vi "iBeam Laser Engine.vi"(0 "iBeam Laser Notifier":string, 11 "COM Port":string[](array[string])) -> ()   [LabVIEW 2016]
uses:
  Laser Controls/Laser Notifier Element.ctl
  Laser Controls/Laser Actions.ctl
  Laser Controls/Laser Settings.ctl
  Laser Controls/Laser Parameters.ctl
  Laser Controls/Laser Status.ctl
  <vilib>/Instr/_visa.llb/VISA Configure Serial Port (Instr).vi
panel:
  in  "Get Status":bool
  in  "Get Power":bool
  out "Laser Status":string
  out "Power (uW)":string
  out "Startup Error":errorcluster
  in  "Quit":bool
  in  "Enable Ext":bool
  in  "Laser Power (mW)":dbl
  in  "Laser On/Off":bool
  out "Serial Number":string
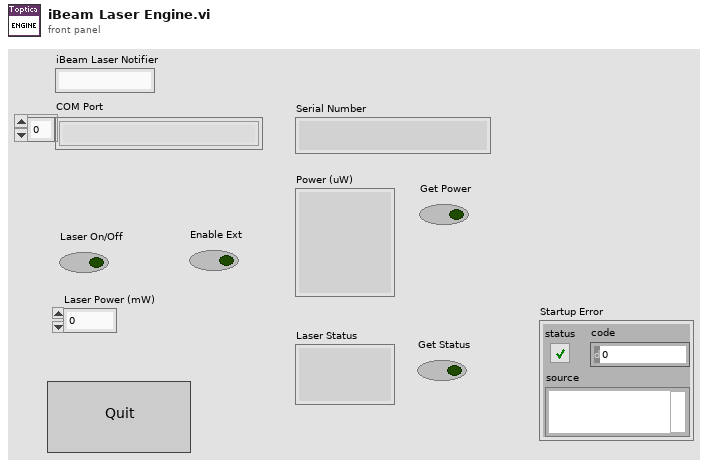
[diagram p1: front panel]
types:
  T1 = typedef "Laser Notifier Element.ctl" = cluster{"Laser Action":T2, "Received?":bool, "Enabled (Interlock)?":bool, "Light Emission?":bool, "Power (mW)":dbl, "Settings":T3, "Status":T5, "Error":errorcluster}
  T2 = typedef "Laser Actions.ctl" = enum16{"Error Check", "Set On/Off", "Set Power", "Set Parameter", "Get Power", "Get Status", "Get Parameter", "Quit"}
  T3 = typedef "Laser Settings.ctl" = cluster{"Laser Parameters":T4, "Value":dbl}
  T4 = typedef "Laser Parameters.ctl" = enum16{"Wavelength (nm)", "Pulsing?", "Rep. Rate", "External Control"}
  T5 = typedef "Laser Status.ctl" = enum16{"Warmup", "Ready", "Emission", "Tuning", "Error"}
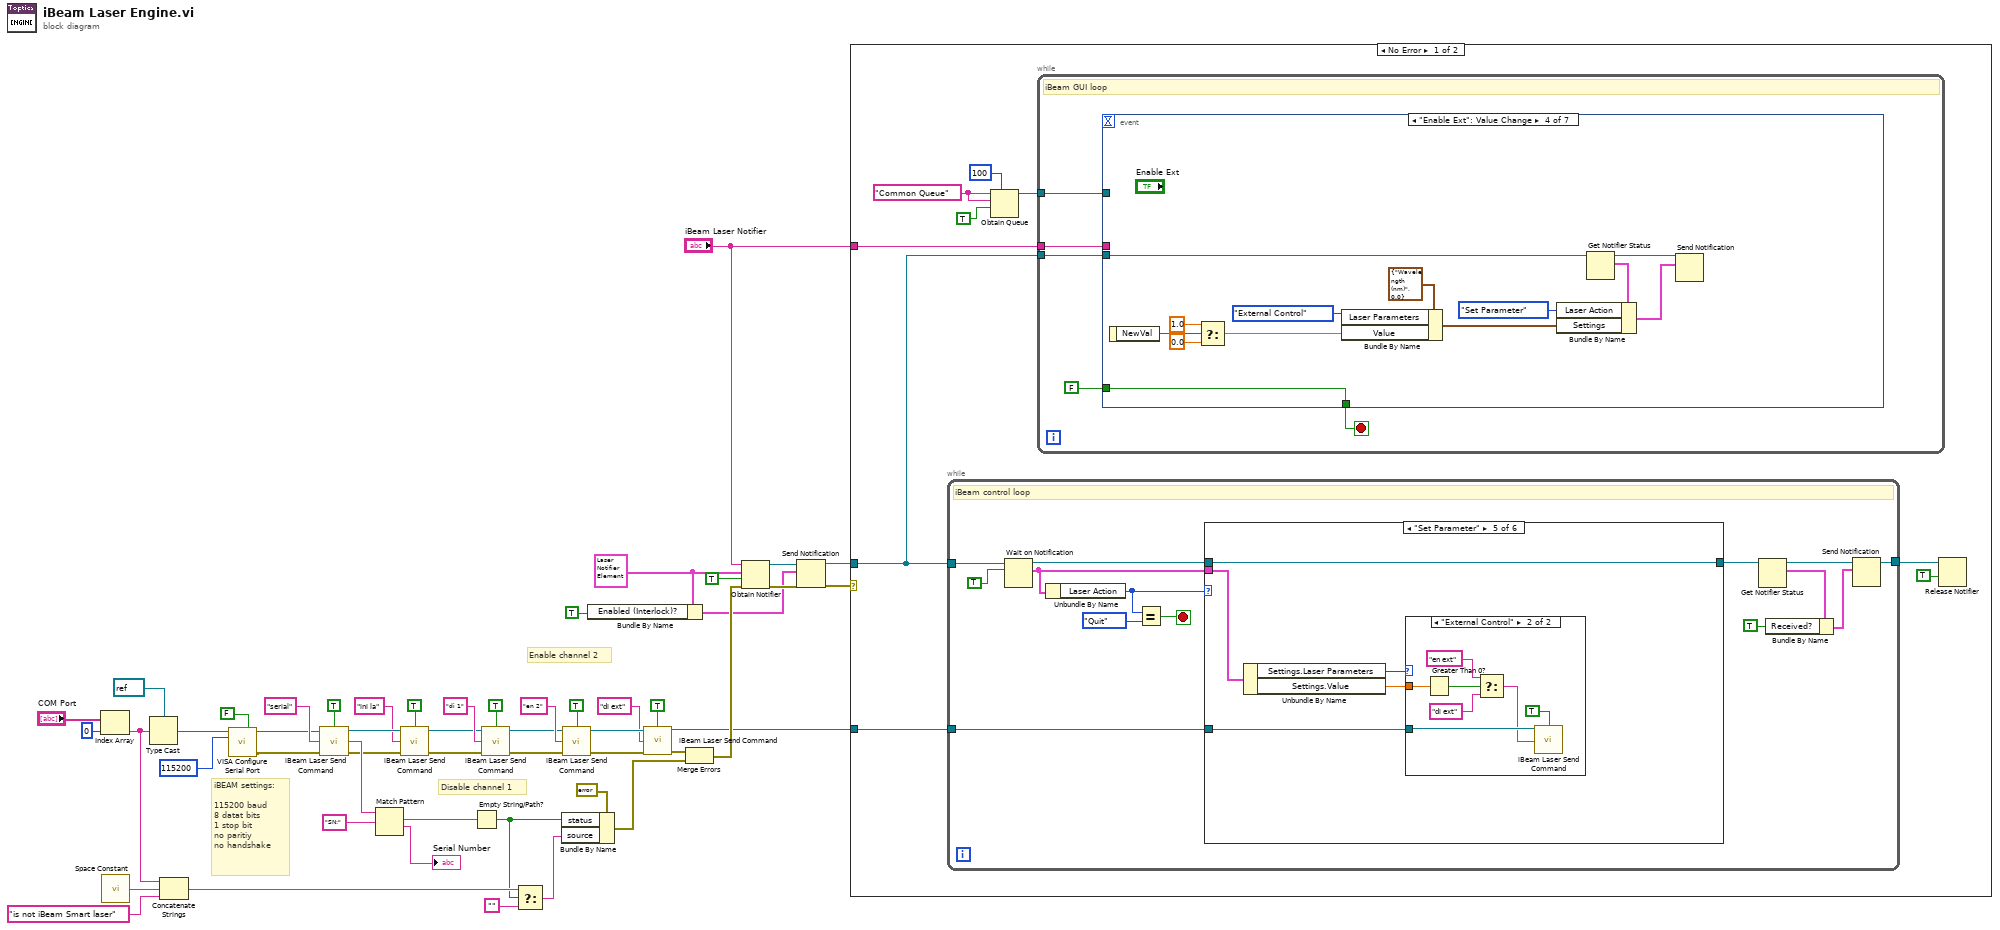
[diagram p0: block diagram]
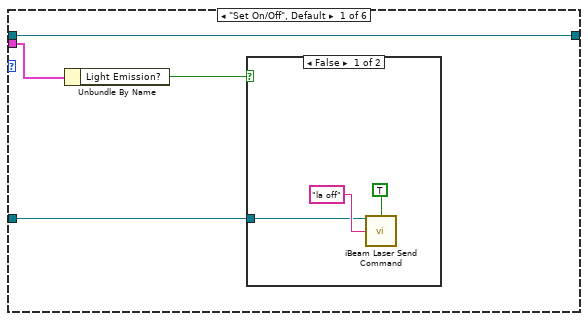
[diagram p2: hidden frame]
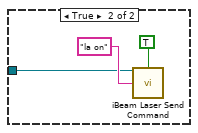
[diagram p3: hidden frame]
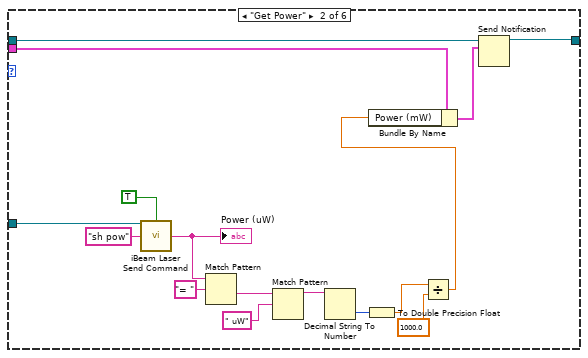
[diagram p4: hidden frame]
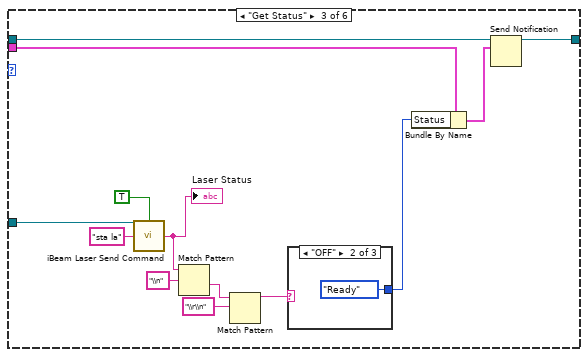
[diagram p5: hidden frame]
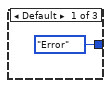
[diagram p6: hidden frame]
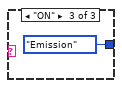
[diagram p7: hidden frame]
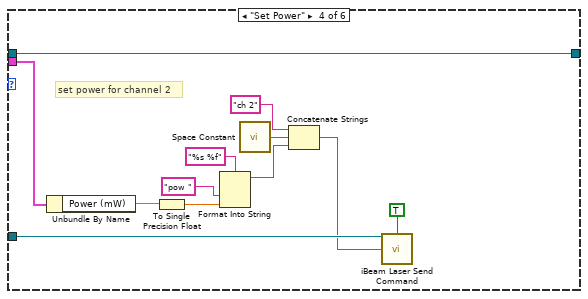
[diagram p8: hidden frame]
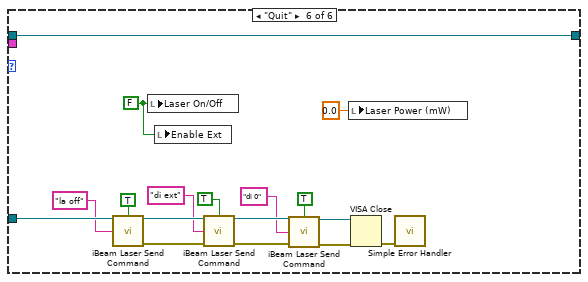
[diagram p10: hidden frame]
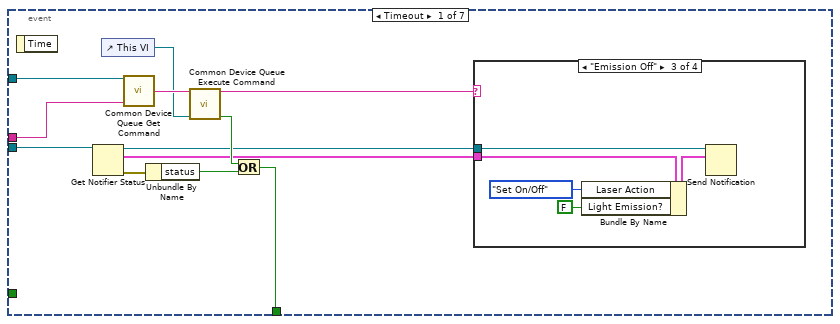
[diagram p11: hidden frame]
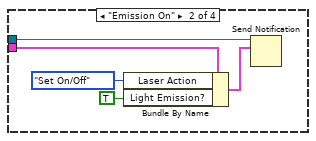
[diagram p13: hidden frame]
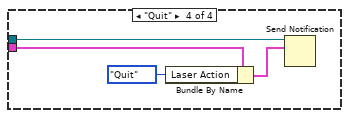
[diagram p14: hidden frame]
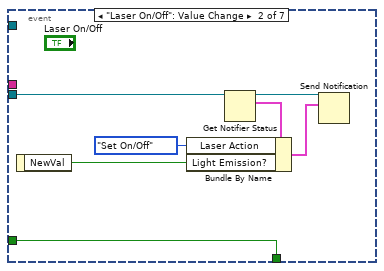
[diagram p15: hidden frame]
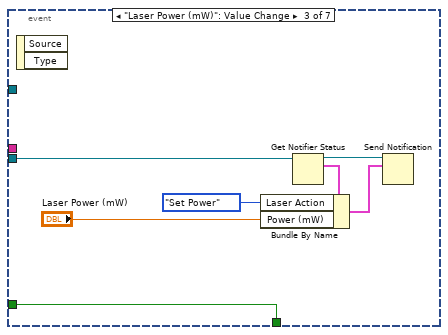
[diagram p16: hidden frame]
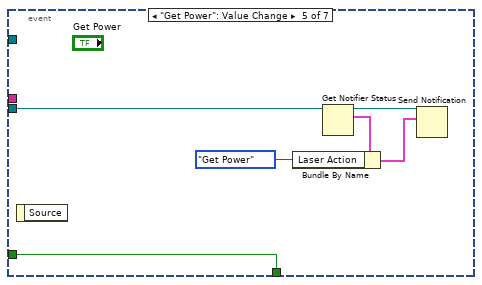
[diagram p17: hidden frame]
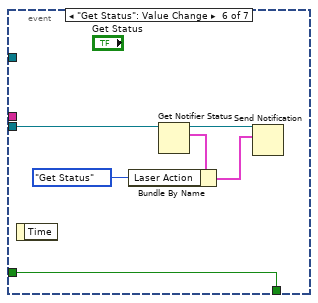
[diagram p18: hidden frame]
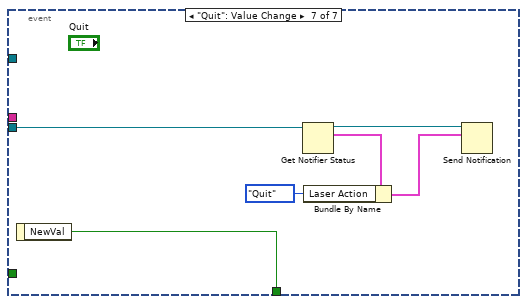
[diagram p19: hidden frame]
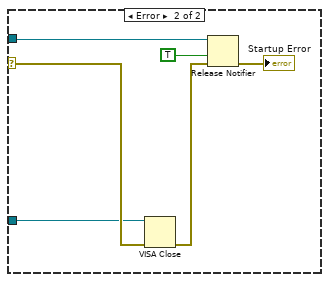
[diagram p20: hidden frame]
diagram:
  w14 = T1 {"Laser Action"=enum."Set On/Off", "Received?"=FALSE, "Enabled (Interlock)?"=FALSE, "Light Emission?"=FALSE, "Power (mW)"=0.0, "Settings"={"Laser Parameters"=enum."Wavelength (nm)", "Value"=0.0}, "Status"=enum."Error", "Error"={"status"=FALSE, "code"=0, "source"=""}} ("Laser Notifier Element")
  # "iBEAM settings:\n\n115200 baud\n8 datat bits\n1 stop bit\nno paritiy\nno handshake"
  # "Enable channel 2"
  # "Disable channel 1"
  n1 = Index Array(array="COM Port", index=0) -> (element=w44:string)
  n2 = call <vilib>:"Space Constant.vi"() -> ("String"=w43:string)
  n3 = Type Cast(type=refnum<visa-resource-name> refnum ("VISA resource name"), x=w44) -> (*(type *) &x=w3:refnum<visa-resource-name>)
  n4 = Concatenate Strings(w44, w43, "is not iBeam Smart laser" ("string")) -> (w40:string)
  n5 = call-poly "VISA Configure Serial Port"("VISA resource name"=w3, "Enable Termination\nChar (T)"=FALSE ("Enable Termination\nChar (T)"), "baud rate (9600)"=u32 115200 ("baud rate (115200)")) -> ("VISA resource name out"=w2:refnum<visa-resource-name>, "error out"=w1:errorcluster)  [unwired: 11 in]
  n6 = call "iBeam Laser Send Command.vi"("VISA Ref"=w2, "Wait for Reply?"=TRUE, "Command"="serial" ("command"), "Error In"=w1) -> ("VISA Ref Out"=w30:refnum<visa-resource-name>, "Response"=w47:string, "Error Out"=w29:errorcluster)  [unwired: 9 in]
  n7 = Match Pattern(string=w47, regular expression="SN:") -> (match substring=w41:string, after substring=→"Serial Number":string)  [unwired: 1 in, 2 out]
  n8 = call "iBeam Laser Send Command.vi"("VISA Ref"=w30, "Wait for Reply?"=TRUE, "Command"="ini la", "Error In"=w29) -> ("VISA Ref Out"=w22:refnum<visa-resource-name>, "Error Out"=w21:errorcluster)  [unwired: 9 in, 1 out]
  n9 = Empty String/Path?(string/path=w41) -> (empty?=w37:bool)
  n10 = call "iBeam Laser Send Command.vi"("VISA Ref"=w22, "Wait for Reply?"=TRUE, "Command"="di 1", "Error In"=w21) -> ("VISA Ref Out"=w19:refnum<visa-resource-name>, "Error Out"=w18:errorcluster)  [unwired: 9 in, 1 out]
  n11 = Select(t=w40, s=w37, f="") -> (s? t:f=w36:string)
  n12 = Bundle By Name(cluster=errorcluster {"status"=FALSE, "code"=0, "source"=""} ("error in"), "status"=w37, "source"=w36) -> (w35:errorcluster)
  n13 = call "iBeam Laser Send Command.vi"("VISA Ref"=w19, "Wait for Reply?"=TRUE, "Command"="en 2", "Error In"=w18) -> ("VISA Ref Out"=w11:refnum<visa-resource-name>, "Error Out"=w8:errorcluster)  [unwired: 9 in, 1 out]
  n14 = Bundle By Name(cluster=w14, "Enabled (Interlock)?"=TRUE) -> (w12:T1)
  n15 = call "iBeam Laser Send Command.vi"("VISA Ref"=w11, "Wait for Reply?"=TRUE, "Command"="di ext", "Error In"=w8) -> ("VISA Ref Out"=w10:refnum<visa-resource-name>, "Error Out"=w7:errorcluster)  [unwired: 9 in, 1 out]
  n16 = Merge Errors(w7, w35) -> (w34:errorcluster)
  n17 = Obtain Notifier(name (unnamed)="iBeam Laser Notifier", notification data type=w14, create if not found? (T)=TRUE, error in (no error)=w34) -> (notifier out=w24:refnum<notifier>, error out=w33:errorcluster)  [unwired: 1 out]
  n18 = Send Notification(notification=w12, notifier=w24, error in (no error)=w33) -> (notifier out=w26:refnum<notifier>, error out=w32:errorcluster)
  n19 = case shown="No Error" w32 {
    selector: w32 -> [_ w235]
    tunnel: w26 -> [w60 w236]
    tunnel: w10 -> [w59 w234]
    tunnel: "iBeam Laser Notifier" -> [w53 _]
    frame No Error {
      w56 = "Common Queue" ("Unique Notifier Name")
      n20 = while {
        tunnel: w60 -> [w74]
        tunnel: w59 -> [w70]
        tunnel: [w62] -> w57
        stop <- w73 stop-if-true
        # "iBeam control loop"
        n21 = Wait on Notification(notifier=w74, ignore previous (F)=TRUE) -> (notifier out=w69:refnum<notifier>, notification=w71:T1)  [unwired: 2 in, 2 out]
        n22 = Unbundle By Name(w71) -> ("Laser Action"=w72:T2)
        n23 = Equal?(x=w72, y=Laser_Actions."Quit") -> (x = y?=w73:bool)
        n24 = case shown="\"Set Parameter\"" w72 {
          tunnel: w71 -> [w78 w89 w105 w128 w133 _]
          tunnel: w70 -> [w76 w100 w113 w123 w132 w157]
          tunnel: w69 -> [w75 w87 w102 w119 w131 w141]
          tunnel: [w75 w86 w101 w119 w131 w141] -> w67
          frame "Set On/Off", Default {
            n25 = Unbundle By Name(w78) -> ("Light Emission?"=w77:bool)
            n26 = case shown="False" w77 {
              tunnel: w76 -> [w79 w82]
              frame False {
                n27 = call "iBeam Laser Send Command.vi"("VISA Ref"=w79, "Wait for Reply?"=TRUE, "Command"="la off" ("command")) -> ()  [unwired: 10 in, 3 out]
              }
              frame True {
                n28 = call "iBeam Laser Send Command.vi"("VISA Ref"=w82, "Wait for Reply?"=TRUE, "Command"="la on" ("command")) -> ()  [unwired: 10 in, 3 out]
              }
            }
          }
          frame "Get Power" {
            n29 = call "iBeam Laser Send Command.vi"("VISA Ref"=w100, "Wait for Reply?"=TRUE, "Command"="sh pow") -> ("Response"=w97:string)  [unwired: 10 in, 2 out]
            "Power (uW)" <- w97
            n30 = Match Pattern(string=w97, regular expression="= ") -> (after substring=w95:string)  [unwired: 1 in, 3 out]
            n31 = Match Pattern(string=w95, regular expression=" uW") -> (before substring=w93:string)  [unwired: 1 in, 3 out]
            n32 = Decimal String To Number(string=w93) -> (number=w92:i32)  [unwired: 2 in, 1 out]
            n33 = To Double Precision Float(number=w92) -> (double precision float=w91:dbl)
            n34 = Divide(x=w91, y=1000.0) -> (x/y=w85:dbl)
            n35 = Bundle By Name(cluster=w89, "Power (mW)"=w85) -> (w88:T1)
            n36 = Send Notification(notification=w88, notifier=w87) -> (notifier out=w86:refnum<notifier>)  [unwired: 1 in, 1 out]
          }
          frame "Get Status" {
            n37 = call "iBeam Laser Send Command.vi"("VISA Ref"=w113, "Wait for Reply?"=TRUE, "Command"="sta la") -> ("Response"=w110:string)  [unwired: 10 in, 2 out]
            "Laser Status" <- w110
            n38 = Match Pattern(string=w110, regular expression="\\n") -> (after substring=w109:string)  [unwired: 1 in, 3 out]
            n39 = Match Pattern(string=w109, regular expression="\\r\\n") -> (before substring=w106:string)  [unwired: 1 in, 3 out]
            n40 = case shown="\"OFF\"" w106 {
              tunnel: [Laser_Status."Error" ("Status") Laser_Status."Ready" ("Status") Laser_Status."Emission" ("Status")] -> w104
              frame Default {
              }
              frame "OFF" {
              }
              frame "ON" {
              }
            }
            n41 = Bundle By Name(cluster=w105, "Status"=w104) -> (w103:T1)
            n42 = Send Notification(notification=w103, notifier=w102) -> (notifier out=w101:refnum<notifier>)  [unwired: 1 in, 1 out]
          }
          frame "Set Power" {
            # "set power for channel 2"
            n43 = Unbundle By Name(w128) -> ("Power (mW)"=w118:dbl)
            n44 = To Single Precision Float(number=w118) -> (single precision float=w117:sgl)
            n45 = Format Into String(format string="%s %f", "pow " ("string"), w117) -> (resulting string=w124:string)  [unwired: 2 in, 1 out]
            n46 = call <vilib>:"Space Constant.vi"() -> ("String"=w125:string)
            n47 = Concatenate Strings("ch 2" ("string"), w125, w124) -> (w122:string)
            n48 = call "iBeam Laser Send Command.vi"("VISA Ref"=w123, "Wait for Reply?"=TRUE, "Command"=w122) -> ()  [unwired: 10 in, 3 out]
          }
          frame "Set Parameter" {
            n49 = Unbundle By Name(w133) -> ("Settings.Laser Parameters"=w130:T4, "Settings.Value"=w129:dbl)
            n50 = case shown="\"External Control\"" w130 {
              tunnel: w132 -> [_ w140]
              tunnel: w129 -> [_ w138]
              frame Default {
              }
              frame "External Control" {
                n51 = Greater Than 0?(x=w138) -> (x > 0?=w137:bool)
                n52 = Select(t="en ext" ("Command"), s=w137, f="di ext" ("Command")) -> (s? t:f=w134:string)
                n53 = call "iBeam Laser Send Command.vi"("VISA Ref"=w140, "Wait for Reply?"=TRUE, "Command"=w134) -> ()  [unwired: 10 in, 3 out]
              }
            }
          }
          frame "Quit" {
            w143 = FALSE ("Laser On/Off")
            n54 = call "iBeam Laser Send Command.vi"("VISA Ref"=w157, "Wait for Reply?"=TRUE, "Command"="la off") -> ("VISA Ref Out"=w155:refnum<visa-resource-name>, "Error Out"=w154:errorcluster)  [unwired: 10 in, 1 out]
            n55 = local write "Laser On/Off"(w143) -> ()
            n56 = local write "Enable Ext"(w143) -> ()
            n57 = call "iBeam Laser Send Command.vi"("VISA Ref"=w155, "Wait for Reply?"=TRUE, "Command"="di ext", "Error In"=w154) -> ("VISA Ref Out"=w149:refnum<visa-resource-name>, "Error Out"=w148:errorcluster)  [unwired: 9 in, 1 out]
            n58 = call "iBeam Laser Send Command.vi"("VISA Ref"=w149, "Wait for Reply?"=TRUE, "Command"="di 0", "Error In"=w148) -> ("VISA Ref Out"=w147:refnum<visa-resource-name>, "Error Out"=w146:errorcluster)  [unwired: 9 in, 1 out]
            n59 = local write "Laser Power (mW)"(sgl 0.0 ("Laser Power (mW)")) -> ()
            n60 = VISA Close(VISA resource name=w147, error in (no error)=w146) -> (error out=w152:errorcluster)
            n61 = call <vilib>:"Simple Error Handler.vi"("error in (no error)"=w152) -> ()  [unwired: 4 in, 5 out]
          }
        }
        n62 = Get Notifier Status(notifier=w67) -> (notifier out=w64:refnum<notifier>, current notification=w66:T1)  [unwired: 1 in, 3 out]
        n63 = Bundle By Name(cluster=w66, "Received?"=TRUE) -> (w63:T1)
        n64 = Send Notification(notification=w63, notifier=w64) -> (notifier out=w62:refnum<notifier>)  [unwired: 1 in, 1 out]
      }
      n65 = Obtain Queue(max queue size (-1, unlimited)=100, name (unnamed)=w56, element data type=w56, create if not found? (T)=TRUE) -> (queue out=w52:refnum<queue>)  [unwired: 1 in, 2 out]
      n66 = while {
        tunnel: w60 -> [w162]
        tunnel: w53 -> [w159]
        tunnel: w52 -> [w158]
        stop <- w160 stop-if-true
        # "iBeam GUI loop"
        n67 = event shown="[3] \"Enable Ext\": Value Change" {
          selector: _ -> [_ _ _ _ _ _ _]
          dyn-events: _ -> [_ _ _ _ _ _ _]
          timeout: _ -> [_ _ _ _ _ _ _]
          tunnel: w162 -> [w169 w195 w202 w215 w218 w223 w231]
          tunnel: FALSE ("stop") -> [_ w190 w198 w211 w216 w222 _]
          tunnel: [w165 w190 w198 w211 w216 w222 w233] -> w160
          tunnel: w159 -> [w173 _ _ _ _ _ _]
          tunnel: w158 -> [w174 _ _ _ _ _ _]
          event Timeout {
            n68 = event-data() -> ()  [unwired: 1 in, 1 out]
            n69 = Get Notifier Status(notifier=w169) -> (notifier out=w164:refnum<notifier>, current notification=w163:T1, error out=w168:errorcluster)  [unwired: 1 in, 2 out]
            n70 = control-ref of="This VI"() -> (w171:refnum<vi>)
            n71 = call "Common Device Queue Get Command.vi"("Common Queue"=w174, "Notifier Name"=w173) -> ("Command"=w172:string)  [unwired: 12 in, 1 out]
            n72 = Unbundle By Name(w168) -> ("status"=w166:bool)
            n73 = call "Common Device Queue Execute Command.vi"("Common Command"=w172, "VI Refnum"=w171) -> ("Common Command"=w170:string, "Quit?"=w167:bool)  [unwired: 12 in]
            n74 = Or(x=w167, y=w166) -> (x .or. y?=w165:bool)
            n75 = case shown="\"Emission Off\"" w170 {
              tunnel: w164 -> [_ w179 w182 w187]
              tunnel: w163 -> [_ w178 w181 w186]
              frame Default {
              }
              frame "Emission On" {
                n76 = Bundle By Name(cluster=w178, "Laser Action"=Laser_Actions."Set On/Off", "Light Emission?"=TRUE) -> (w177:T1)
                n77 = Send Notification(notification=w177, notifier=w179) -> ()  [unwired: 1 in, 2 out]
              }
              frame "Emission Off" {
                n78 = Bundle By Name(cluster=w181, "Laser Action"=Laser_Actions."Set On/Off", "Light Emission?"=FALSE) -> (w183:T1)
                n79 = Send Notification(notification=w183, notifier=w182) -> ()  [unwired: 1 in, 2 out]
              }
              frame "Quit" {
                n80 = Bundle By Name(cluster=w186, "Laser Action"=Laser_Actions."Quit") -> (w188:T1)
                n81 = Send Notification(notification=w188, notifier=w187) -> ()  [unwired: 1 in, 2 out]
              }
            }
          }
          event "Laser On/Off": Value Change {
            n82 = event-data() -> ("NewVal"=w193:bool)  [unwired: 1 in]
            n83 = Get Notifier Status(notifier=w195) -> (notifier out=w194:refnum<notifier>, current notification=w191:T1)  [unwired: 1 in, 3 out]
            n84 = Bundle By Name(cluster=w191, "Laser Action"=Laser_Actions."Set On/Off", "Light Emission?"=w193) -> (w192:T1)
            n85 = Send Notification(notification=w192, notifier=w194) -> ()  [unwired: 1 in, 2 out]
          }
          event "Laser Power (mW)": Value Change {
            n86 = event-data() -> ()  [unwired: 1 in, 2 out]
            n87 = Get Notifier Status(notifier=w202) -> (notifier out=w200:refnum<notifier>, current notification=w201:T1)  [unwired: 1 in, 3 out]
            n88 = Bundle By Name(cluster=w201, "Laser Action"=Laser_Actions."Set Power", "Power (mW)"="Laser Power (mW)") -> (w199:T1)
            n89 = Send Notification(notification=w199, notifier=w200) -> ()  [unwired: 1 in, 2 out]
          }
          event "Enable Ext": Value Change {
            n90 = event-data() -> ("NewVal"=w206:bool)  [unwired: 1 in]
            n91 = Select(t=1.0, s=w206, f=0.0) -> (s? t:f=w203:dbl)
            n92 = Bundle By Name(cluster=T3 {"Laser Parameters"=enum."Wavelength (nm)", "Value"=0.0} ("Settings"), "Laser Parameters"=Laser_Parameters."External Control", "Value"=w203) -> (w208:T3)
            n93 = Get Notifier Status(notifier=w215) -> (notifier out=w213:refnum<notifier>, current notification=w214:T1)  [unwired: 1 in, 3 out]
            n94 = Bundle By Name(cluster=w214, "Laser Action"=Laser_Actions."Set Parameter", "Settings"=w208) -> (w212:T1)
            n95 = Send Notification(notification=w212, notifier=w213) -> ()  [unwired: 1 in, 2 out]
          }
          event "Get Power": Value Change {
            n96 = event-data() -> ()  [unwired: 1 in, 1 out]
            n97 = Get Notifier Status(notifier=w218) -> (notifier out=w221:refnum<notifier>, current notification=w220:T1)  [unwired: 1 in, 3 out]
            n98 = Bundle By Name(cluster=w220, "Laser Action"=Laser_Actions."Get Power") -> (w217:T1)
            n99 = Send Notification(notification=w217, notifier=w221) -> ()  [unwired: 1 in, 2 out]
          }
          event "Get Status": Value Change {
            n100 = event-data() -> ()  [unwired: 1 in, 1 out]
            n101 = Get Notifier Status(notifier=w223) -> (notifier out=w227:refnum<notifier>, current notification=w226:T1)  [unwired: 1 in, 3 out]
            n102 = Bundle By Name(cluster=w226, "Laser Action"=Laser_Actions."Get Status") -> (w224:T1)
            n103 = Send Notification(notification=w224, notifier=w227) -> ()  [unwired: 1 in, 2 out]
          }
          event "Quit": Value Change {
            n104 = event-data() -> ("NewVal"=w233:bool)  [unwired: 1 in]
            n105 = Get Notifier Status(notifier=w231) -> (notifier out=w232:refnum<notifier>, current notification=w230:T1)  [unwired: 1 in, 3 out]
            n106 = Bundle By Name(cluster=w230, "Laser Action"=Laser_Actions."Quit") -> (w229:T1)
            n107 = Send Notification(notification=w229, notifier=w232) -> ()  [unwired: 1 in, 2 out]
          }
        }
      }
      n108 = Release Notifier(notifier=w57, force destroy? (F)=TRUE) -> ()  [unwired: 1 in, 3 out]
    }
    frame Error {
      n109 = VISA Close(VISA resource name=w234, error in (no error)=w235) -> (error out=w238:errorcluster)
      n110 = Release Notifier(notifier=w236, force destroy? (F)=TRUE, error in (no error)=w238) -> (error out=→"Startup Error":errorcluster)  [unwired: 2 out]
    }
  }
